vi "LS330_OpenFile.vi"() -> (0 "error out":errorcluster, 1 "file or folder exists?":bool, 3 "File RefOut":refnum<file>)   [LabVIEW 2021]
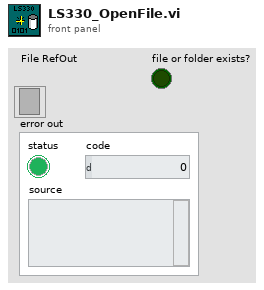
[diagram p1: front panel]
types:
  T1 = enum16{"open", "replace", "create", "open or create", "replace or create", "replace or create with confirmation"}
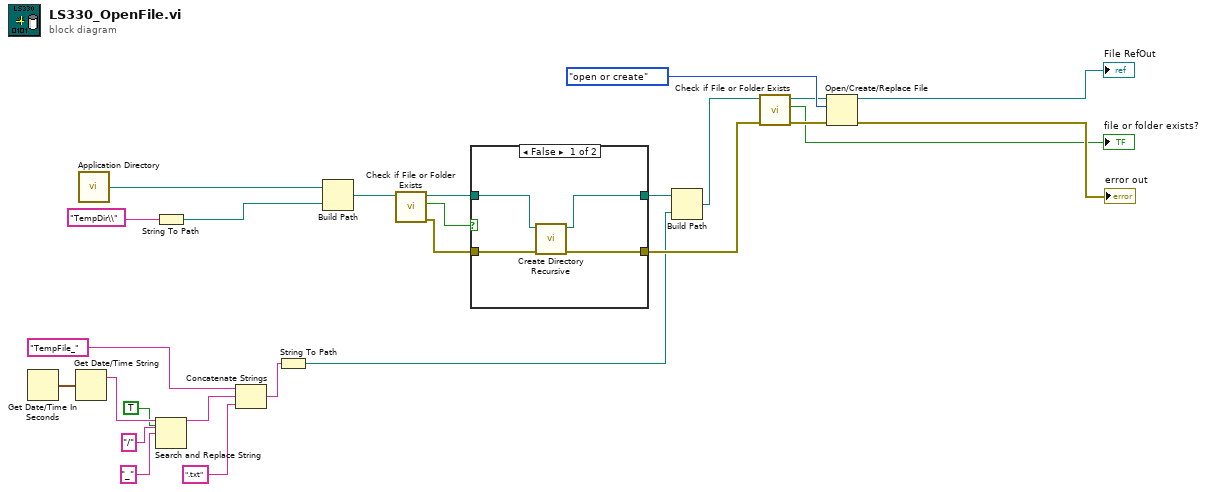
[diagram p0: block diagram]
diagram:
  n1 = Get Date/Time In Seconds() -> (seconds since 1Jan1904=w26:timestamp)
  n2 = Get Date/Time String(seconds (now)=w26) -> (date string=w25:string)  [unwired: 2 in, 1 out]
  n3 = call <vilib>:"Application Directory.vi"() -> ("Application Directory"=w11:path)
  n4 = String To Path(string="TempDir\\") -> (path=w9:path)
  n5 = Search and Replace String(replace all?=TRUE ("replace all? (F)"), input string=w25, search string="/", replace string="_" ("replace string (\"\")")) -> (result string=w21:string)  [unwired: 4 in, 3 out]
  n6 = Concatenate Strings("TempFile_" ("string"), w21, ".txt" ("string")) -> (w20:string)
  n7 = String To Path(string=w20) -> (path=w1:path)
  n8 = Build Path(base path=w11, name or relative path=w9) -> (appended path=w8:path)
  n9 = call <vilib>:"Check if File or Folder Exists.vi"("path"=w8) -> ("error out"=w5:errorcluster, "file or folder exists?"=w6:bool, "dup path"=w7:path)  [unwired: 8 in]
  n10 = case shown="False" w6 {
    tunnel: w7 -> [w28 w32]
    tunnel: w5 -> [w30 w31]
    tunnel: [w27 w32] -> w3
    tunnel: [w29 w31] -> w4
    frame False {
      n11 = call <vilib>:"Create Directory Recursive.vi"("error in (no error)"=w30, "directory"=w28) -> ("error out"=w29:errorcluster, "directory copy"=w27:path)  [unwired: 3 in, 1 out]
    }
    frame True {
    }
  }
  n12 = Build Path(base path=w3, name or relative path=w1) -> (appended path=w2:path)
  n13 = call <vilib>:"Check if File or Folder Exists.vi"("error in (no error)"=w4, "path"=w2) -> ("error out"=w14:errorcluster, "file or folder exists?"=→"file or folder exists?":bool, "dup path"=w15:path)  [unwired: 7 in]
  n14 = Open/Create/Replace File(file path (use dialog)=w15, error in=w14, operation (0:open)=T1."open or create") -> (refnum out=→"File RefOut":refnum<file>, error out=→"error out":errorcluster)  [unwired: 3 in, 1 out]
